vi "test Set ObjectType_1.vi"(11 "Test Case In":refnum<class "test Electronic Datasheet.lvclass">) -> (0 "error out":errorcluster, 3 "Test Case Out":refnum<class "test Electronic Datasheet.lvclass">)   [LabVIEW 2024, in "test Electronic Datasheet.lvclass"]
uses:
  test Electronic Datasheet.lvclass
  C:/Program Files/National Instruments/LabVIEW 2025/vi.lib/Astemes/LUnit/Test Case.lvclass
  Core/Object Type/Object Type Base.lvclass
  <vilib>/Astemes/LUnit/Test Case.lvclass/Test Case.ctl
  Core/Value/Value.lvclass
  <vilib>/Astemes/LUnit/Test Case.lvclass
  Core/Object Type.ctl
  Core/Electronic Datasheet.lvlib
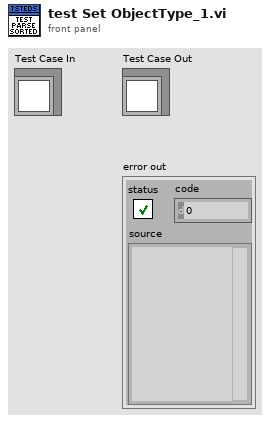
[diagram p1: front panel]
types:
  T1 = typedef "Electronic Datasheet.lvlib/Object Type.ctl" = u8
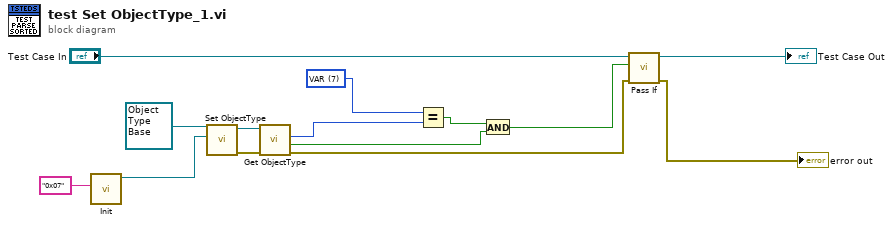
[diagram p0: block diagram]
diagram:
  w1 = T1 7 items=["NULL"=0, "DOMAIN"=2, "DEFTYPE"=5, "DEFSTRUCT"=6, "VAR"=7, "ARRAY"=8, "RECORD"=9] ("ObjectType")
  n1 = call "Init.vi"("Value"="0x07") -> ("Value out"=w10:refnum<class "Value.lvclass">)  [unwired: 9 in, 1 out]
  n2 = call-dynamic "Set ObjectType.vi"("ObjectType"=w10, "Object Type in"=refnum<class "Object Type Base.lvclass"> refnum ("EDS.lvlib:Object Type.lvclass")) -> ("error out"=w8:errorcluster, "Object Type out"=w5:refnum<class "Object Type Base.lvclass">)  [unwired: 8 in]
  n3 = call-dynamic "Get ObjectType.vi"("error in"=w8, "Object Type in"=w5) -> ("error out"=w6:errorcluster, "Defined?"=w2:bool, "ObjectType"=w7:T1)  [unwired: 6 in, 1 out]
  n4 = Equal?(x=w1, y=w7) -> (x = y?=w3:bool)
  n5 = And(x=w3, y=w2) -> (x .and. y?=w4:bool)
  n6 = call <vilib>:"Pass If.vi"("error in (no error)"=w6, "Pass?"=w4, "LUnit Test Case In"="Test Case In") -> ("error out"=→"error out":errorcluster, "LUnit Test Case Out"=→"Test Case Out":refnum<class "test Electronic Datasheet.lvclass">)  [unwired: 7 in]
